vi "Rinocloud_HTTP_ancestors_to_tree.vi"(4 "error in (no error)":errorcluster, 6 "id":string, 7 "Tree Ref in":refnum<vi>) -> (0 "error out":errorcluster, 1 "Status":T1={"headers"="", "body"="", "ID"="", "Saved"=TRUE}, 2 "last ID":string, 3 "Tree Ref out":refnum<vi>)   [LabVIEW 2011, in "Rinocloud Library.lvlib"]
uses:
  Rinocloud Library.lvlib
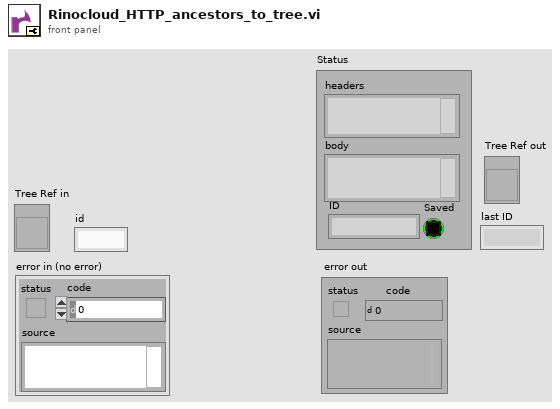
[diagram p1: front panel]
types:
  T1 = cluster{"headers":string, "body":string, "ID":string, "Saved":bool}
  T2 = cluster{"id":string, "name":string, "created_on":string, "updated_on":string, "tags":string, "notes":string, "record type":string, "metadata (JSON)":string}[]
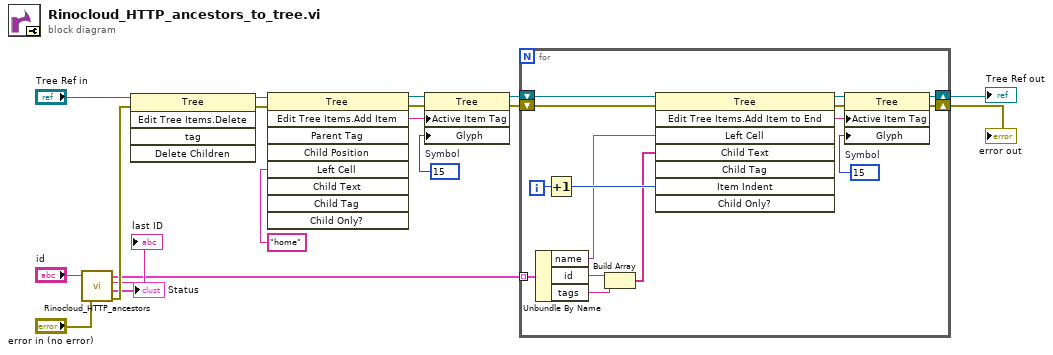
[diagram p0: block diagram]
diagram:
  w17 = 15  # Symbol
  n1 = call "Rinocloud_HTTP_ancestors.vi"("error in (no error)"="error in (no error)", "id"="id") -> ("error out"=w6:errorcluster, "Status"=→"Status":T1, "last ID"=→"last ID":string, "metadata array"=w4:T2)  [unwired: 2 in]
  n2 = invoke class="Tree" method="Edit Tree Items.Delete"(reference="Tree Ref in", error in=w6) -> (reference out=w11:refnum<vi>, error out=w12:errorcluster)  [unwired: 3 in, 3 out]
  n3 = invoke class="Tree" method="Edit Tree Items.Add Item"(reference=w11, error in=w12, "Left Cell"="home" ("Left Cell String")) -> (reference out=w14:refnum<vi>, error out=w15:errorcluster, "Edit Tree Items:Add Item"=w16:string)  [unwired: 6 in, 6 out]
  n4 = property class="Tree"(reference=w14, error in=w15, "Active Item Tag"=w16, "Glyph"=w17) -> (reference out=w8:refnum<vi>, error out=w7:errorcluster)
  n5 = for {
    shift-right: [w28] -> w3
    shift-left: w8 -> [w29]
    shift-right: [w26] -> w2
    shift-left: w7 -> [w27]
    tunnel: w4 -> [w23] mode=indexing
    i -> [w24]
    w33 = 15  # Symbol
    n6 = Unbundle By Name(w23) -> ("name"=w22:string, "id"=w21:string, "tags"=w20:string)
    n7 = Increment(x=w24) -> (x+1=w25:i32)
    n8 = Build Array(w21, w20) -> (w19:string[])
    n9 = invoke class="Tree" method="Edit Tree Items.Add Item to End"(reference=w29, error in=w27, "Left Cell"=w22, "Child Text"=w19, "Item Indent"=w25) -> (reference out=w30:refnum<vi>, error out=w31:errorcluster, "Edit Tree Items:Add Item to End"=w32:string)  [unwired: 3 in, 5 out]
    n10 = property class="Tree"(reference=w30, error in=w31, "Active Item Tag"=w32, "Glyph"=w33) -> (reference out=w28:refnum<vi>, error out=w26:errorcluster)
  }
  "error out" <- w2
  "Tree Ref out" <- w3
